vi "NotifyObserver_Array.vi"(8 "error in":errorcluster, 9 "ObservableDataValue":variant[](array[variant]), 10 "ObservableDataName":string[](array[string]), 11 "IstanceName":string) -> (0 "error out":errorcluster)   [LabVIEW 2025, in "ObserverClass.lvlib"]
doc: "Send Notification to all the Observer"
uses:
  ObserverClass.lvlib
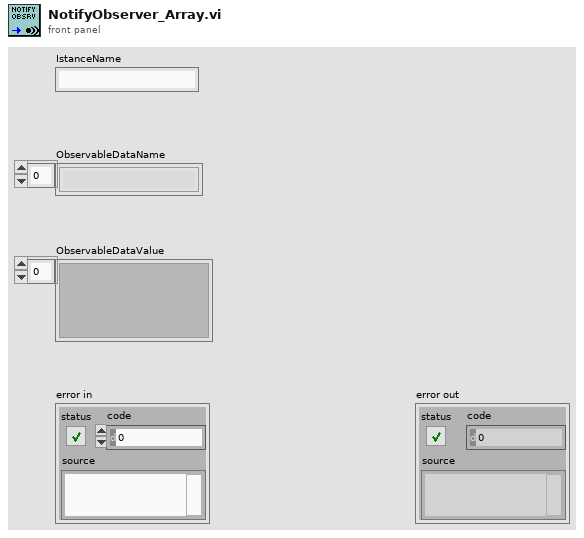
[diagram p1: front panel]
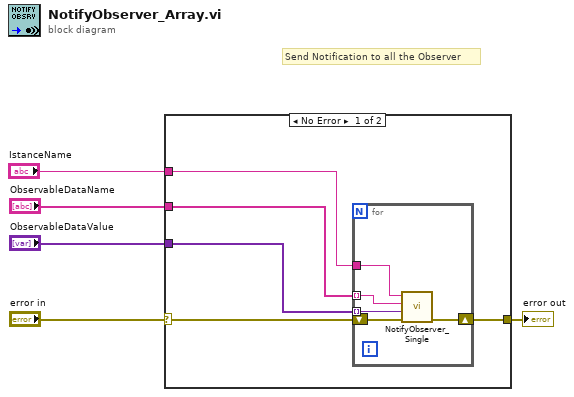
[diagram p0: block diagram]
diagram:
  # "Send Notification to all the Observer"
  n1 = case shown="No Error" "error in" {
    selector: "error in" -> [w10 w16]
    tunnel: "ObservableDataName" -> [w8 _]
    tunnel: "ObservableDataValue" -> [w6 _]
    tunnel: "IstanceName" -> [w7 _]
    tunnel: [w9 w16] -> w5
    frame No Error {
      n2 = for {
        tunnel: w8 -> [w12] mode=indexing
        tunnel: w7 -> [w11]
        tunnel: w6 -> [w13] mode=indexing
        shift-right: [w14] -> w9
        shift-left: w10 -> [w15]
        n3 = call "NotifyObserver_Single.vi"("error in"=w15, "ObservableDataValue"=w13, "ObservableDataName"=w12, "IstanceName"=w11) -> ("error out"=w14:errorcluster)  [unwired: 7 in]
      }
    }
    frame Error {
    }
  }
  "error out" <- w5
